vi "CMN_GetFromCmdLine.vi"(10 "str in":string) -> (2 "str out":string)   [LabVIEW 2016]
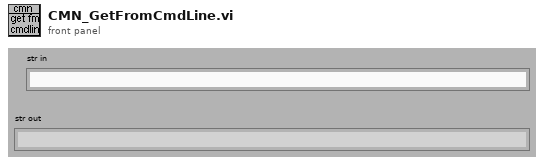
[diagram p1: front panel]
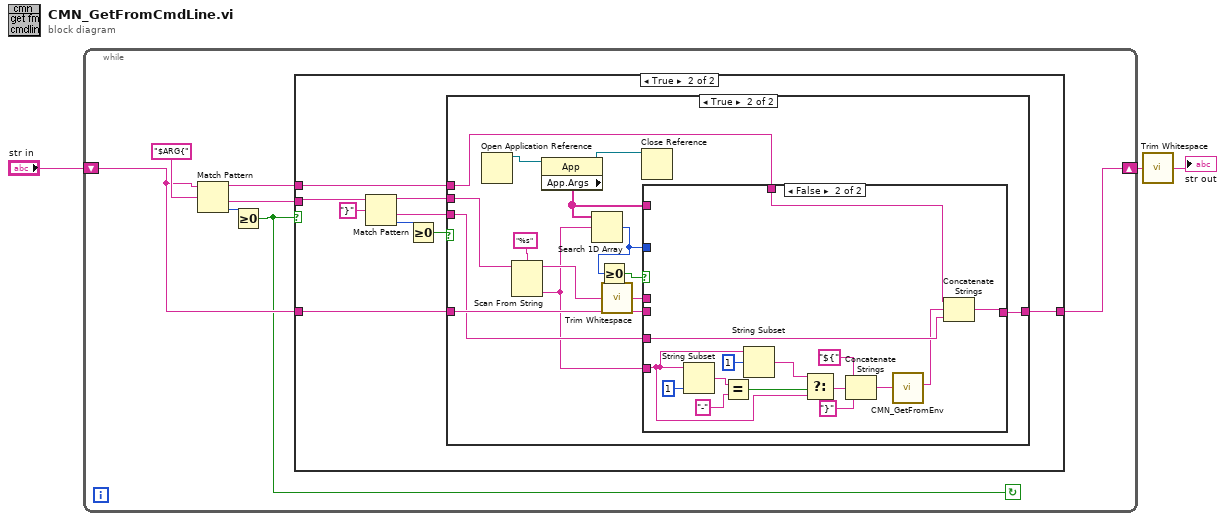
[diagram p0: block diagram]
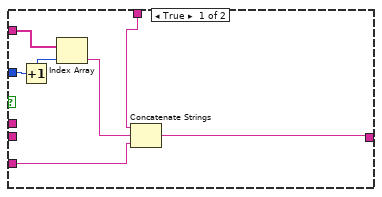
[diagram p4: hidden frame]
diagram:
  n1 = while {
    shift-right: [w4] -> w2
    shift-left: "str in" -> [w6]
    stop <- w5 continue-if-true
    n2 = Match Pattern(string=w6, regular expression="$ARG{" ("x")) -> (before substring=w7:string, after substring=w8:string, offset past match=w10:i32)  [unwired: 2 out]
    n3 = Greater Or Equal To 0?(x=w10) -> (x >= 0?=w5:bool)
    n4 = case shown="True" w5 {
      tunnel: w6 -> [w11 w16]
      tunnel: [w11 w15] -> w4
      tunnel: w8 -> [_ w20]
      tunnel: w7 -> [_ w13]
      frame False {
      }
      frame True {
        n5 = Match Pattern(string=w20, regular expression="}") -> (before substring=w14:string, after substring=w12:string, offset past match=w18:i32)  [unwired: 2 out]
        n6 = Greater Or Equal To 0?(x=w18) -> (x >= 0?=w17:bool)
        n7 = case shown="True" w17 {
          tunnel: w16 -> [w21 w30]
          tunnel: [w21 w29] -> w15
          tunnel: w14 -> [_ w33]
          tunnel: w13 -> [_ w24]
          tunnel: w12 -> [_ w23]
          frame False {
          }
          frame True {
            n8 = Open Application Reference() -> (3:w35:refnum<vi>)  [unwired: 1 in, 4 out]
            n9 = Scan From String(format string="%s", input string=w33) -> (remaining string=w28:string, output 1=w22:string)  [unwired: 2 in, 3 out]
            n10 = property class="App"(reference=w35) -> (reference out=w34:refnum<vi>, "App.Args"=w25:string[])  [unwired: 1 in, 1 out]
            n11 = Search 1D Array(1D array=w25, element=w22) -> (index of element=w26:i32)  [unwired: 1 out]
            n12 = Greater Or Equal To 0?(x=w26) -> (x >= 0?=w31:bool)
            n13 = call <vilib>:"Trim Whitespace.vi"("string"=w28) -> ("trimmed string"=w27:string)  [unwired: 1 in]
            n14 = Close Reference(reference=w34) -> ()  [unwired: 1 in, 1 out]
            n15 = case shown="False" w31 {
              tunnel: w30 -> [_ _]
              tunnel: [w37 w56] -> w29
              tunnel: w27 -> [_ _]
              tunnel: w26 -> [w41 _]
              tunnel: w25 -> [w42 _]
              tunnel: w24 -> [w38 w57]
              tunnel: w23 -> [w36 w55]
              tunnel: w22 -> [_ w50]
              frame True {
                n16 = Increment(x=w41) -> (x+1=w40:i32)
                n17 = Index Array(array=w42, index=w40) -> (element=w39:string)
                n18 = Concatenate Strings(w38, w39, w36) -> (w37:string)
              }
              frame False {
                n19 = String Subset(string=w50, length (rest)=1 ("length (rest)")) -> (substring=w53:string)  [unwired: 1 out]
                n20 = Equal?(x=w53, y="-") -> (x = y?=w51:bool)
                n21 = String Subset(string=w50, offset (0)=1) -> (substring=w48:string)  [unwired: 1 out]
                n22 = Select(t=w48, s=w51, f=w50) -> (s? t:f=w47:string)
                n23 = Concatenate Strings("${" ("string"), w47, "}" ("string")) -> (w44:string)
                n24 = call "CMN_GetFromEnv.vi"("str in"=w44) -> ("str out"=w43:string)  [unwired: 10 out]
                n25 = Concatenate Strings(w57, w43, w55) -> (w56:string)
              }
            }
          }
        }
      }
    }
  }
  n26 = call <vilib>:"Trim Whitespace.vi"("string"=w2) -> ("trimmed string"=→"str out":string)  [unwired: 1 in]
